vi "Find Best Cost.vi"(11 "State":cluster{"Hallway":string[], "Rooms":string[][]}) -> (3 "Best Cost":u64)   [LabVIEW 2019, in "23.lvlib"]
uses:
  23.lvlib
  LRU Queue.vi
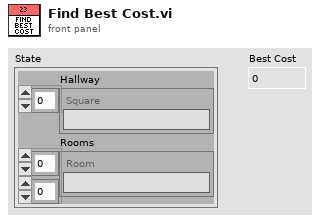
[diagram p1: front panel]
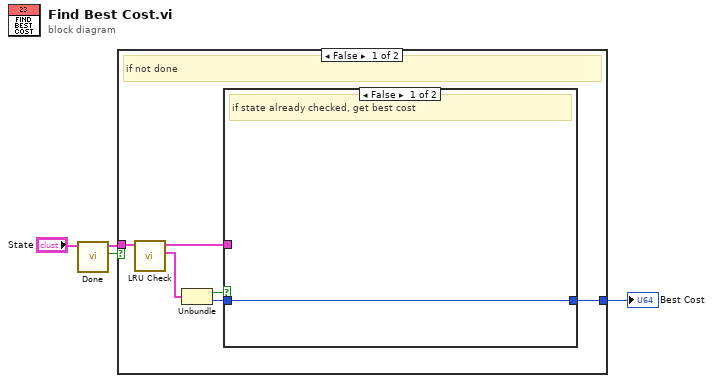
[diagram p0: block diagram]
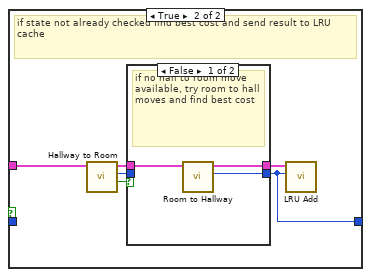
[diagram p2: hidden frame]
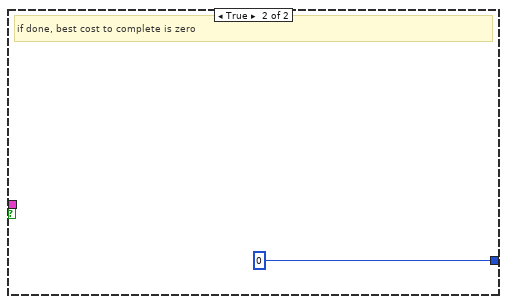
[diagram p4: hidden frame]
diagram:
  n1 = call "Done.vi"("State in"="State") -> ("Done?"=w3:bool, "State out"=w2:cluster{"Hallway":string[], "Rooms":string[][]})  [unwired: 9 in]
  n2 = case shown="False" w3 {
    tunnel: [w8 u64 0] -> w1
    tunnel: w2 -> [w7 _]
    frame False {
      # "if not done"
      n3 = call "LRU Check.vi"("State in"=w7) -> ("LRU Check Result"=w6:cluster{"Key Not Found?":bool, "Value":u64}, "State out"=w5:cluster{"Hallway":string[], "Rooms":string[][]})  [unwired: 9 in]
      n4 = Unbundle(w6) -> ("Key Not Found?"=w10:bool, "Value"=w9:u64)
      n5 = case shown="False" w10 {
        tunnel: w9 -> [w11 _]
        tunnel: [w11 w14] -> w8
        tunnel: w5 -> [_ w12]
        frame False {
          # "if state already checked, get best cost"
        }
        frame True {
          # "if state not already checked find best cost and send result to LRU cache"
          n6 = call "Hallway to Room.vi"("State in"=w12) -> ("Moved?"=w17:bool, "Best Cost"=w16:u64, "State out"=w15:cluster{"Hallway":string[], "Rooms":string[][]})  [unwired: 8 in]
          n7 = case shown="False" w17 {
            tunnel: w16 -> [_ w22]
            tunnel: [w20 w22] -> w14
            tunnel: w15 -> [w19 w21]
            tunnel: [w18 w21] -> w13
            frame False {
              # "if no hall to room move available, try room to hall moves and find best cost"
              n8 = call "Room to Hallway.vi"("State in"=w19) -> ("Best Cost"=w20:u64, "State out"=w18:cluster{"Hallway":string[], "Rooms":string[][]})  [unwired: 9 in]
            }
            frame True {
              # "if moved from hall to room return best cost"
            }
          }
          n9 = call "LRU Add.vi"("Value"=w14, "State"=w13) -> ()  [unwired: 10 in]
        }
      }
    }
    frame True {
      # "if done, best cost to complete is zero"
    }
  }
  "Best Cost" <- w1
